vi "Set Send Header.vi"(8 "error in (no error)":errorcluster, 9 "Value":string, 10 "Name":string, 11 "WebSockets in":refnum<class "WebSocket.lvclass">) -> (0 "error out":errorcluster, 3 "WebSockets out":refnum<class "WebSocket.lvclass">)   [LabVIEW 2013, in "WebSockets.lvlib" / "WebSocket.lvclass"]
doc: "Sets a send header to send from the WebSocket connection to the corresponding endpoint."
uses:
  WebSocket.lvclass
  WebSocket.lvclass/WebSocket.ctl
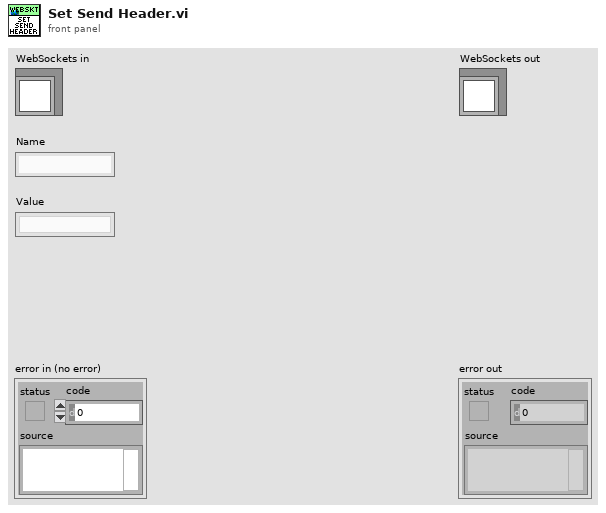
[diagram p1: front panel]
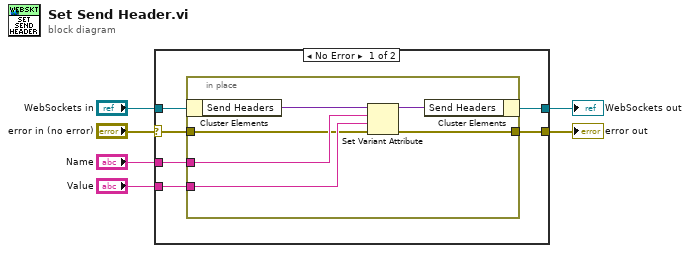
[diagram p0: block diagram]
diagram:
  n1 = case shown="No Error" "error in (no error)" {
    selector: "error in (no error)" -> [w8 w20]
    tunnel: [w7 w20] -> w5
    tunnel: [w11 w19] -> w3
    tunnel: "WebSockets in" -> [w12 w19]
    tunnel: "Name" -> [w10 _]
    tunnel: "Value" -> [w9 _]
    frame No Error {
      n2 = in-place {
        in-place-border: w10 -> [w16]
        in-place-border: w9 -> [w15]
        in-place-border: w8 -> [w14]
        in-place-border: [w13] -> w7
        n3 = in-place-cluster #1(w12) -> ("Send Headers"=w18:variant)
        n4 = Set Variant Attribute(Variant=w18, name=w16, value=w15, error in=w14) -> (Variant out=w17:variant, error out=w13:errorcluster)  [unwired: 1 out]
        n5 = in-place-cluster #1("Send Headers"=w17) -> (w11:refnum<class "WebSocket.lvclass">)
      }
    }
    frame Error {
    }
  }
  "error out" <- w5
  "WebSockets out" <- w3
